vi "Requests.vi"(8 "error in (no error)":errorcluster, 9 "write enable":bool=TRUE, 11 "SMSD in":refnum<class "SMSD.lvclass">) -> (0 "error out":errorcluster, 3 "SMSD out":refnum<class "SMSD.lvclass">)   [LabVIEW 2021, in "SMSD.lvclass"]
uses:
  SMSD.lvclass
  D:/my_projects/projects/Algorithms/Labview/21/Modbus/MB_TCP2/MB_TCP.lvclass
  Ctl/ERROR_OR_COMMANT_Type.ctl
  SMSD.lvclass/SMSD.ctl
  MB_TCP.lvclass/MB_TCP.ctl
  NI_modbus_upd/TCP/TCP.lvclass/TCP.ctl
  SMSD_cmd_format.vi
  NI_modbus_upd/TCP/Protocol Read.vi
  NI_modbus_upd/TCP/Protocol Write.vi
  Data Access/Read TCP.vi
  SMSD_cmd_Data_format.vi
  SMSD_LAN_COMMAND.vi
  <vilib>/Utility/error.llb/Clear Errors.vi
  NI_modbus_upd/TCP/TCP.lvclass
  ICPCON Registers/ICPCON Registers.lvlib
  MB_TCP.lvclass
panel:
  out "position":i32
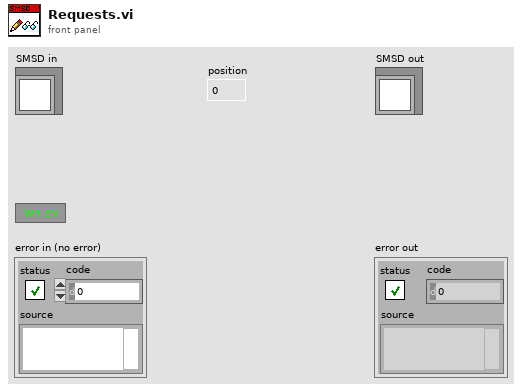
[diagram p1: front panel]
types:
  T1 = enum8{"CMD_PowerSTEP01_END", "CMD_PowerSTEP01_GET_SPEED", "CMD_PowerSTEP01_STATUS_IN_EVENT", "CMD_PowerSTEP01_SET_MODE", "CMD_PowerSTEP01_GET_MODE", "CMD_PowerSTEP01_SET_MIN_SPEED", "CMD_PowerSTEP01_SET_MAX_SPEED", "CMD_PowerSTEP01_SET_ACC", "CMD_PowerSTEP01_SET_DEC", "CMD_PowerSTEP01_SET_FS_SPEED", "CMD_PowerSTEP01_SET_MASK_EVENT", "CMD_PowerSTEP01_GET_ABS_POS", "CMD_PowerSTEP01_GET_EL_POS", "CMD_PowerSTEP01_GET_STATUS_AND_CLR", "CMD_PowerSTEP01_RUN_F", "CMD_PowerSTEP01_RUN_R", "CMD_PowerSTEP01_MOVE_F", "CMD_PowerSTEP01_MOVE_R", "CMD_PowerSTEP01_GO_TO_F", "CMD_PowerSTEP01_GO_TO_R", "CMD_PowerSTEP01_GO_UNTIL_F", "CMD_PowerSTEP01_GO_UNTIL_R", "CMD_PowerSTEP01_SCAN_ZERO_F", "CMD_PowerSTEP01_SCAN_ZERO_R", "CMD_PowerSTEP01_SCAN_LABEL_F", "CMD_PowerSTEP01_SCAN_LABEL_R", "CMD_PowerSTEP01_GO_ZERO", "CMD_PowerSTEP01_GO_LABEL", "CMD_PowerSTEP01_GO_TO", "CMD_PowerSTEP01_RESET_POS", "CMD_PowerSTEP01_RESET_POWERSTEP01", "CMD_PowerSTEP01_SOFT_STOP", "CMD_PowerSTEP01_HARD_STOP", "CMD_PowerSTEP01_SOFT_HI_Z", "CMD_PowerSTEP01_HARD_HI_Z", "CMD_PowerSTEP01_SET_WAIT", "CMD_PowerSTEP01_SET_RELE", "CMD_PowerSTEP01_CLR_RELE", "CMD_PowerSTEP01_GET_RELE", "CMD_PowerSTEP01_WAIT_IN0", "CMD_PowerSTEP01_WAIT_IN1", "CMD_PowerSTEP01_GOTO_PROGRAM", "CMD_PowerSTEP01_GOTO_PROGRAM_IF_IN0", "CMD_PowerSTEP01_GOTO_PROGRAM_IF_IN1", "CMD_PowerSTEP01_LOOP_PROGRAM", "CMD_PowerSTEP01_CALL_PROGRAM", "CMD_PowerSTEP01_RETURN_PROGRAM", "CMD_PowerSTEP01_START_PROGRAM_MEM0", "CMD_PowerSTEP01_START_PROGRAM_MEM1", "CMD_PowerSTEP01_START_PROGRAM_MEM2", "CMD_PowerSTEP01_START_PROGRAM_MEM3", "CMD_PowerSTEP01_STOP_PROGRAM_MEM", "CMD_PowerSTEP01_STEP_CLOCK", "CMD_PowerSTEP01_STOP_USB", "CMD_PowerSTEP01_GET_MIN_SPEED", "CMD_PowerSTEP01_GET_MAX_SPEED", "CMD_PowerSTEP01_GET_STACK", "CMD_PowerSTEP01_GOTO_PROGRAM_IF_ZERO", "CMD_PowerSTEP01_GOTO_PROGRAM_IF_IN_ZERO", "CMD_PowerSTEP01_WAIT_CONTINUE", "CMD_PowerSTEP01_SET_WAIT_2", "CMD_PowerSTEP01_SCAN_MARK2_F", "CMD_PowerSTEP01_SCAN_MARK2_R"}
  T2 = typedef "SMSD.lvclass/ERROR_OR_COMMANT_Type.ctl" = enum8{"OK", "OK_ACCESS", "ERROR_ACCESS", "ERROR_ACCESS_TIMEOUT", "ERROR_XOR", "ERROR_NO_COMMAND", "ERROR_LEN", "ERROR_RANGE", "ERROR_WRITE", "ERROR_READ", "ERROR_PROGRAMS", "ERROR_WRITE_SETUP", "NO_NEXT", "END_PROGRAMS", "COMMAND_GET_STATUS_IN_EVENT", "COMMAND_GET_MODE", "COMMAND_GET_ABS_POS", "COMMAND_GET_EL_POS", "COMMAND_GET_SPEED", "COMMAND_GET_MIN_SPEED", "COMMAND_GET_MAX_SPEED", "COMMAND_GET_STACK", "STATUS_RELE_SET", "STATUS_RELE_CLR"}
  T3 = typedef "ICPCON Registers.lvlib/ICPCON Data.ctl" = cluster{"UTF":refnum<data-value>, "DI":refnum<data-value>, "DW":refnum<data-value>, "DO":refnum<data-value>, "IR":refnum<data-value>, "WR":refnum<data-value>, "OR":refnum<data-value>, "modified":refnum<data-value>}
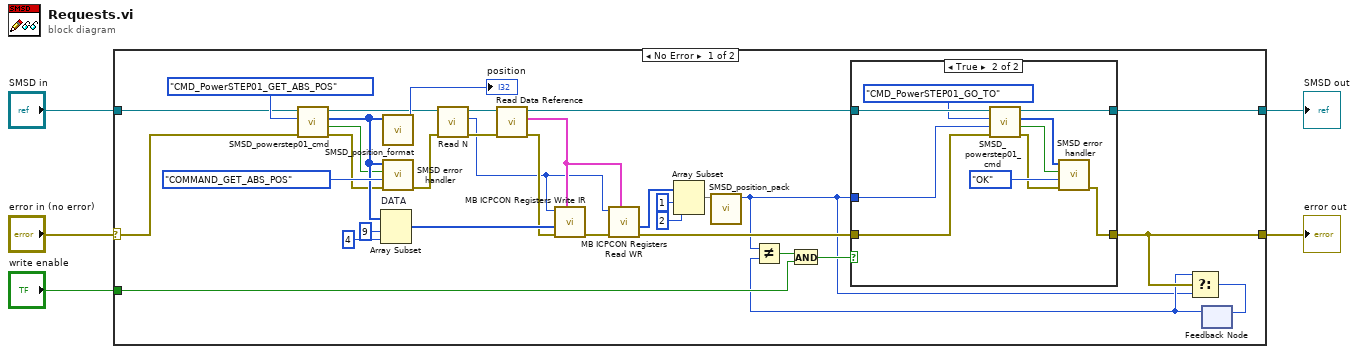
[diagram p0: block diagram]
diagram:
  n1 = case shown="No Error" "error in (no error)" {
    selector: "error in (no error)" -> [w6 w52]
    tunnel: [w23 w52] -> w1
    tunnel: [w33 w51] -> w2
    tunnel: "SMSD in" -> [w10 w51]
    tunnel: "write enable" -> [w25 _]
    frame No Error {
      n2 = call "SMSD_powerstep01_cmd.vi"("error in (no error)"=w6, "COMMAND (END)"=T1."CMD_PowerSTEP01_GET_ABS_POS", "SMSD in"=w10) -> ("error out"=w30:errorcluster, "timed out?"=w28:bool, "data"=w37:u8[], "SMSD out"=w12:refnum<class "SMSD.lvclass">)  [unwired: 5 in]
      n3 = Array Subset "DATA"(array=w37, index=9, length=4) -> (w34:u8[])
      n4 = call "SMSD_position_format.vi"("DATA"=w37) -> ("position"=→"position":i32)  [unwired: 10 in]
      n5 = call "SMSD error handler.vi"("error in (no error)"=w30, "correct answer (OK)"=ERROR_OR_COMMANT_Type."COMMAND_GET_ABS_POS" ("coerced x 2"), "timed out?"=w28, "data"=w37) -> ("error out"=w9:errorcluster)  [unwired: 7 in]
      n6 = call "Read N.vi"("error in (no error)"=w9, "MB_TCP in"=w12) -> ("error out"=w8:errorcluster, "N"=w7:i32, "MB_TCP out"=w11:refnum<class "SMSD.lvclass">)  [unwired: 7 in]
      n7 = call "Read Data Reference.vi"("error in (no error)"=w8, "MB_TCP in"=w11) -> ("error out"=w14:errorcluster, "Data"=w13:T3, "MB_TCP out"=w15:refnum<class "SMSD.lvclass">)  [unwired: 7 in]
      n8 = call "MB ICPCON Registers Write IR.vi"("Data Reference"=w13, "error in (no error)"=w14, "Words In"=w34, "N"=w7) -> ("error out"=w32:errorcluster)  [unwired: 7 in]
      n9 = call "MB ICPCON Registers Read WR.vi"("Data Reference"=w13, "error in (no error)"=w32, "N"=w7) -> ("error out"=w31:errorcluster, "Words out"=w19:u16[])  [unwired: 7 in]
      n10 = Array Subset(array=w19, index=1, length=2) -> (w16:u16[])
      n11 = call "SMSD_position_pack.vi"("DATA"=w16) -> ("position"=w20:u32)  [unwired: 10 in]
      n12 = feedback #1() -> (w22:u32)  [unwired: 1 in]
      n13 = Not Equal?(x=w20, y=w22) -> (x != y?=w26:bool)
      n14 = And(x=w26, y=w25) -> (x .and. y?=w24:bool)
      n15 = case shown="True" w24 {
        tunnel: [w40 w50] -> w33
        tunnel: w15 -> [w40 w49]
        tunnel: [w39 w44] -> w23
        tunnel: w31 -> [w39 w43]
        tunnel: w20 -> [_ w41]
        frame False {
        }
        frame True {
          n16 = call "SMSD_powerstep01_cmd.vi"("error in (no error)"=w43, "DATA (0)"=w41, "COMMAND (END)"=T1."CMD_PowerSTEP01_GO_TO", "SMSD in"=w49) -> ("error out"=w45:errorcluster, "timed out?"=w46:bool, "data"=w48:u8[], "SMSD out"=w50:refnum<class "SMSD.lvclass">)  [unwired: 4 in]
          n17 = call "SMSD error handler.vi"("error in (no error)"=w45, "correct answer (OK)"=ERROR_OR_COMMANT_Type."OK" ("coerced x 2"), "timed out?"=w46, "data"=w48) -> ("error out"=w44:errorcluster)  [unwired: 7 in]
        }
      }
      n18 = Select(t=w22, s=w23, f=w20) -> (s? t:f=w21:u32)
      n19 = feedback-in #1(w21) -> ()
    }
    frame Error {
    }
  }
  "error out" <- w1
  "SMSD out" <- w2
